vi "SVPO Order Metrics for Periodic Inspection (1 Ch).vi"(0 "even-angle signal":cluster{"r0":dbl, "dr":dbl, "Y":dbl[]}={"r0"=0.0, "dr"=1.0, "Y"=[]} {"r0" format="%.2p"; "dr" format="%.2p"; "Y" format="%.2f"}, 1 "update? (T)":bool=TRUE, 2 "reset? (F)":bool, 7 "even-angle position info":T2, 9 "orders":dbl[](array[numeric])=[1.0] format="%.2f", 11 "integration cycles":u32=8, 12 "measurement selection":T1={"speed"=TRUE, "DC gap"=TRUE, "RMS level"=TRUE, "max-min level"=TRUE, "magnitude"=TRUE, "phase"=TRUE}) -> (3 "speed [RPM]":dbl, 4 "DC gap":dbl, 6 "RMS level":dbl, 8 "max-min level":dbl, 10 "magnitudes [RMS]":dbl[](array[numeric]), 15 "phase [phase lag]":dbl[](array[numeric]))   [LabVIEW 2017, in "SoundVib_OrderTracking.lvlib"]
doc: "Computes the metrics of designated orders in an even-angle signal, such as magnitudes, phases, speed, DC gap, RMS level, and max-min level. This VI calculates metrics values from the latest integration cycles of the even-angle signal. Use this VI on embedded targets that have limited computational resources. Wire data to the <B>even-angle signal</B> input to determine the polymorphic instance to use or manually select the instance."
uses:
  <vilib>/addons/Sound and Vibration/Order Analysis/Resample Order Tracking/SoundVib_OrderTracking.lvlib
  <vilib>/addons/Sound and Vibration/Order Analysis/Misc/OAT Position Info.ctl
  <vilib>/Analysis/baseanly.llb/Mean.vi
  <vilib>/Analysis/baseanly.llb/Mean (DBL).vi
  <vilib>/Analysis/5stat.llb/RMS.vi
  <vilib>/Analysis/5stat.llb/RMS (DBL).vi
  <vilib>/addons/Sound and Vibration/Order Analysis/Resample Order Tracking/SubVIs/sv_Buffer Even-Angle Signal (1 Ch).vi
  <vilib>/addons/Sound and Vibration/Order Analysis/Resample Order Tracking/SubVIs/sv_Buffer Specified Cycles.vi
  <vilib>/addons/Sound and Vibration/Order Analysis/Resample Order Tracking/SubVIs/sv_Order Mag and Phase with DFT (N Freq, 1 Ch).vi
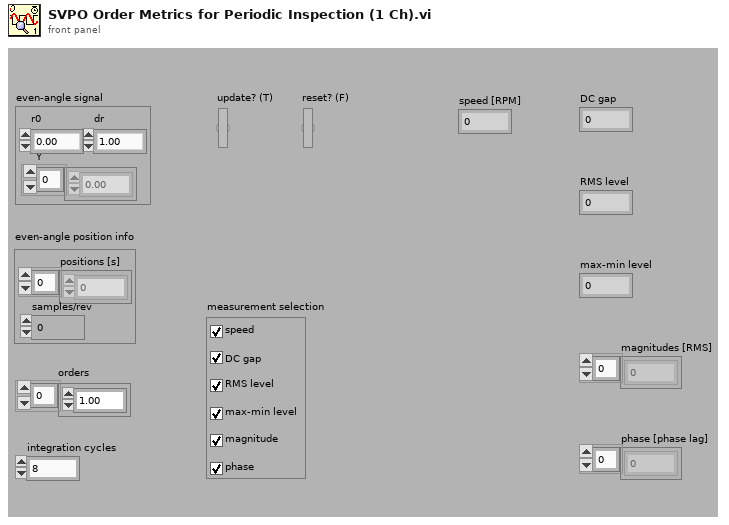
[diagram p1: front panel]
types:
  T1 = cluster{"speed":bool, "DC gap":bool, "RMS level":bool, "max-min level":bool, "magnitude":bool, "phase":bool}
  T2 = typedef "OAT Position Info.ctl" = cluster{"positions [s]":dbl[], "samples/rev":dbl}
  T3 = typedef "svc_Order Metrics State.ctl" = cluster{"buffered signal x[n]":dbl[], "buffered position info x[n]":dbl[]}
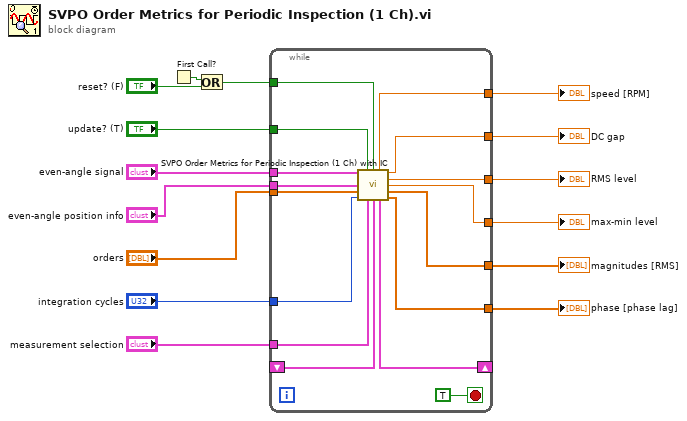
[diagram p0: block diagram]
diagram:
  n1 = First Call?() -> (First Call?: T/F=w14:bool)
  n2 = Or(x=w14, y="reset? (F)") -> (x .or. y?=w11:bool)
  n3 = while {
    tunnel: "even-angle signal" -> [w31]
    tunnel: "update? (T)" -> [w30]
    tunnel: w11 -> [w29]
    tunnel: [w28] -> w10
    tunnel: [w27] -> w9
    tunnel: [w26] -> w8
    tunnel: [w25] -> w7
    tunnel: [w24] -> w6
    tunnel: [w23] -> w5
    tunnel: "integration cycles" -> [w22]
    tunnel: "orders" -> [w21]
    tunnel: "even-angle position info" -> [w20]
    tunnel: "measurement selection" -> [w19]
    shift-right: [w18] -> _
    shift-left: _ -> [w17]
    stop <- TRUE stop-if-true
    n4 = call <vilib>:"SVPO Order Metrics for Periodic Inspection (1 Ch) with IC.vi"("even-angle signal"=w31, "update? (T)"=w30, "reset? (F)"=w29, "even-angle position info"=w20, "orders"=w21, "integration cycles"=w22, "measurement selection"=w19, "initial conditions"=w17) -> ("speed [RPM]"=w28:dbl, "DC gap"=w27:dbl, "RMS level"=w26:dbl, "max-min level"=w25:dbl, "magnitudes [RMS]"=w24:dbl[], "final conditions"=w18:T3, "phase [phase lag]"=w23:dbl[])  [unwired: 1 in]
  }
  "magnitudes [RMS]" <- w6
  "phase [phase lag]" <- w5
  "speed [RPM]" <- w10
  "DC gap" <- w9
  "RMS level" <- w8
  "max-min level" <- w7
